vi "Forno USB.vi"() -> ()   [LabVIEW 2011]
panel:
  out "Manual OFF":bool
  out "Manual ON":bool
  out "Power":dbl(slide) scale=0.0..100.0
  out "Isteresi %":dbl(knob) scale=0.0..10.0
  out "Set Point":dbl(knob) scale=0.0..200.0
  out "Secondi":u8
  out "Minuti":u8
  out "Ora":u8
  in  "Timer ON-OFF":bool
  out "Tempo di funzionamento":cluster{dbl, dbl, dbl}(knob)={0.0, 1.0235355842339904, 13.033095966579117} scale=0.0..60.0
  in  "Secondi":u8(knob) scale=0.0..60.0
  in  "Minuti":u8(knob) scale=0.0..60.0
  in  "Ore":u8(knob) scale=0.0..24.0
  out "Orario":timestamp
  out "Temperatura Interna":dbl(slide) scale=0.0..300.0
  in  "On - Off":bool
  in  "Salvataggio Manuale":bool
  out "File salvato:":path
  in  "Nome File":string
  out "Grafico":cluster{dbl, dbl, dbl, dbl}(graph)
  out "Errore":bool
  out "Forno":bool
  # "DIG-0"
  # "DIG-1"
  # "Analog Channel 9"
  # "Analog Channel  8"
  # "Analog Channel 10"
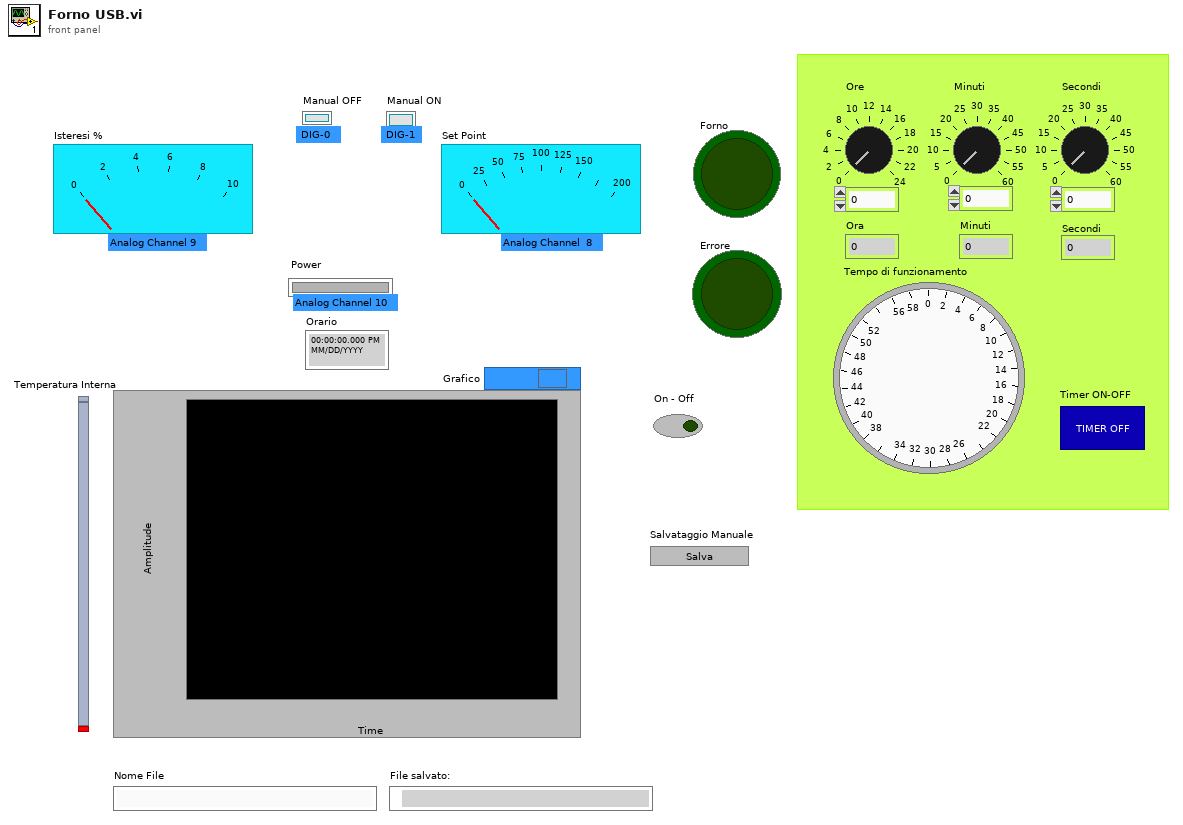
[diagram p1: front panel]
types:
  T1 = enum16{"open", "replace", "create", "open or create", "replace or create", "replace or create with confirmation"}
  T2 = typedef "LVDateTimeRec.ctl" = cluster{"fractional second":dbl, "second":i32, "minute":i32, "hour":i32, "day of month":i32, "month":i32, "year":i32, "day of week":i32, "day of year":i32, "DST":i32}
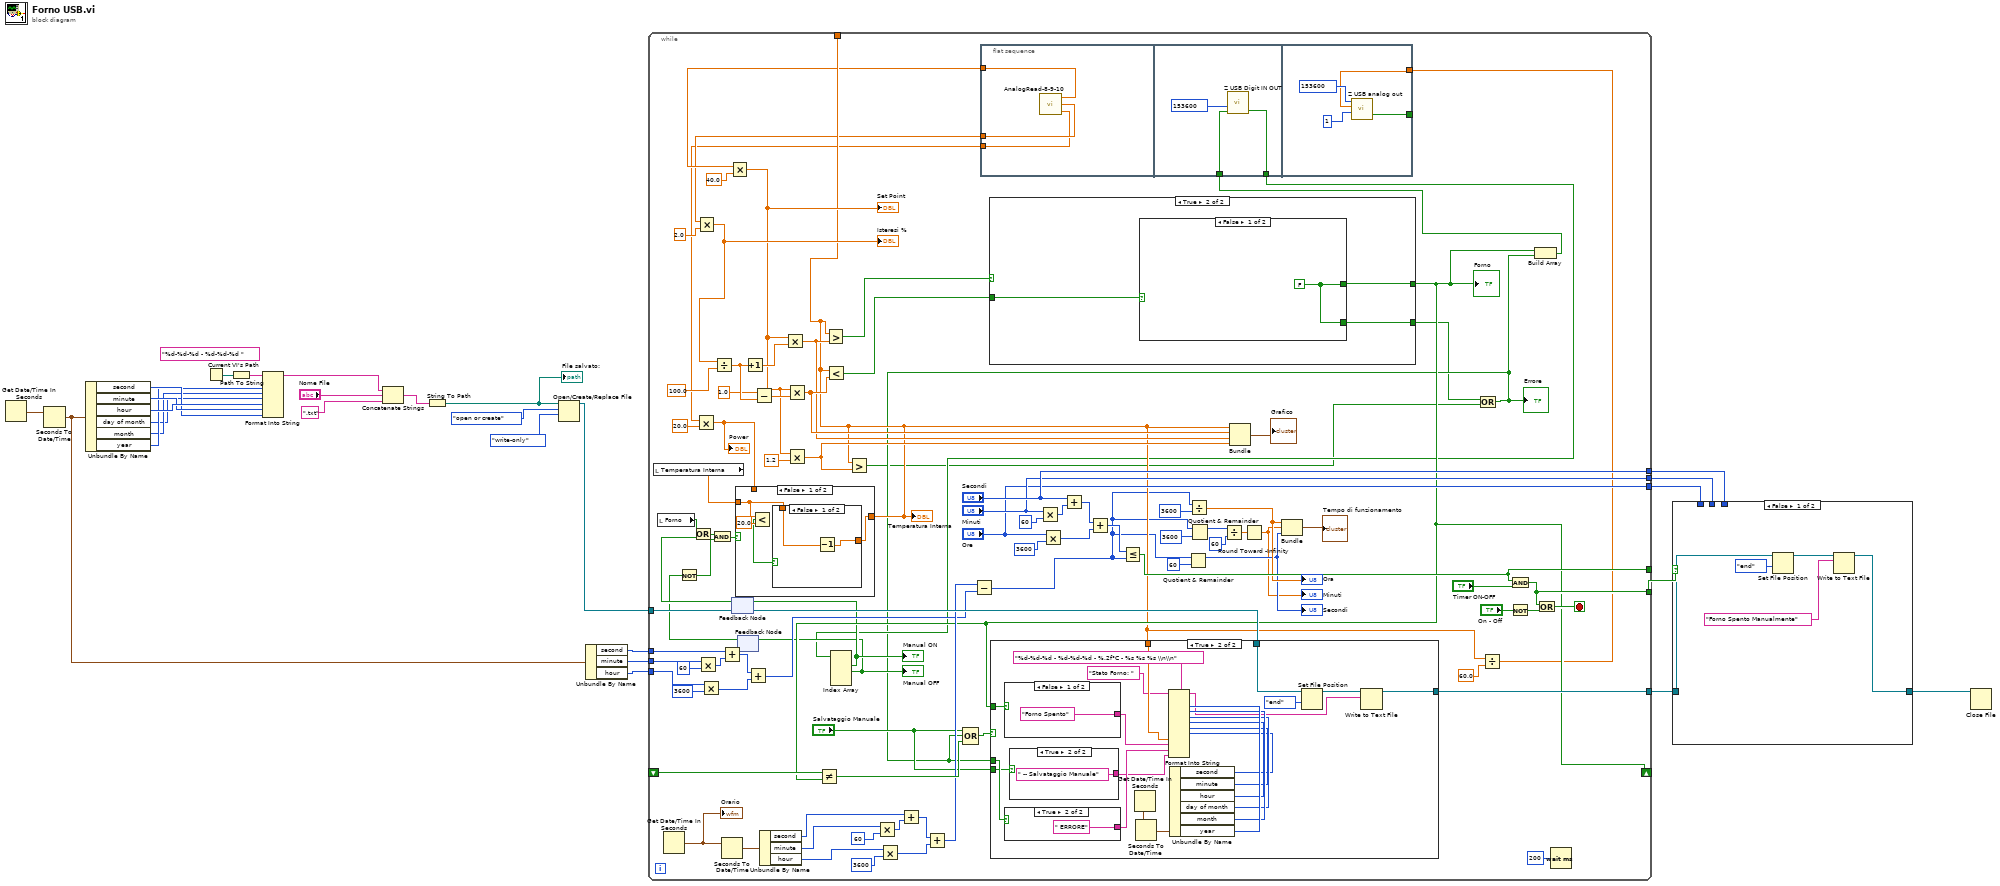
[diagram p0: block diagram]
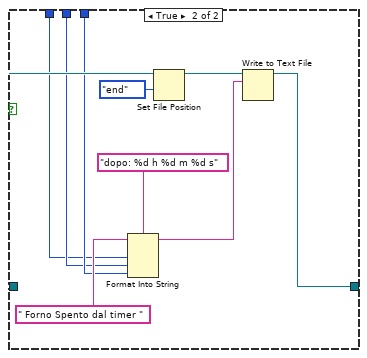
[diagram p2: hidden frame]
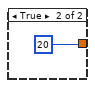
[diagram p3: hidden frame]
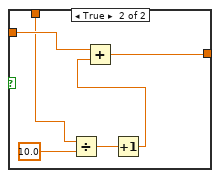
[diagram p4: hidden frame]
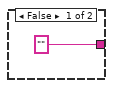
[diagram p6: hidden frame]
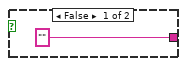
[diagram p7: hidden frame]
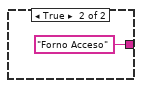
[diagram p8: hidden frame]
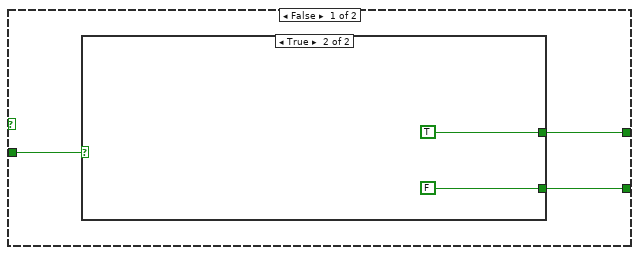
[diagram p9: hidden frame]
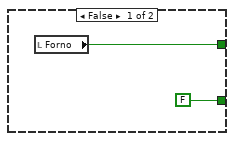
[diagram p10: hidden frame]
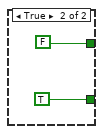
[diagram p11: hidden frame]
diagram:
  (unwired) "%d-%d-%d - %d-%d-%d " ("format string")
  n1 = Get Date/Time In Seconds() -> (seconds since 1Jan1904=w23:timestamp)
  n2 = Seconds To Date/Time(time stamp (now)=w23) -> (date time rec=w12:T2)  [unwired: 1 in]
  n3 = Unbundle By Name(w12) -> ("second"=w20:i32, "minute"=w21:i32, "hour"=w22:i32, "day of month"=w13:i32, "month"=w14:i32, "year"=w15:i32)
  n4 = Current VI's Path() -> (path=w2:path)
  n5 = Path To String(path=w2) -> (string=w1:string)
  n6 = Format Into String(initial string=w1, w15, w14, w13, w22, w21, w20) -> (resulting string=w19:string)  [unwired: 2 in, 1 out]
  n7 = Concatenate Strings(w19, "Nome File", ".txt" ("string")) -> (w25:string)
  n8 = String To Path(string=w25) -> (path=w24:path)
  "File salvato:" <- w24
  n9 = Open/Create/Replace File(file path (use dialog)=w24, operation (0:open)=T1."open or create", access (0:read/write)=enum16{"read/write", "read-only", "write-only"}."write-only") -> (refnum out=w16:refnum<file>)  [unwired: 3 in, 2 out]
  n10 = Unbundle By Name(w12) -> ("second"=w11:i32, "minute"=w10:i32, "hour"=w9:i32)
  n11 = while {
    tunnel: w16 -> [w105]
    tunnel: [w104] -> w8
    tunnel: [w49] -> _
    shift-right: [w55] -> _
    shift-left: _ -> [w100]
    tunnel: w11 -> [w97]
    tunnel: w10 -> [w96]
    tunnel: w9 -> [w93]
    tunnel: [w69] -> _
    tunnel: ["Secondi"] -> w6
    tunnel: ["Minuti"] -> w5
    tunnel: ["Ore"] -> w4
    tunnel: [w67] -> w3
    stop <- w74 stop-if-true
    n12 = local read "Temperatura Interna"() -> (w102:dbl)
    n13 = local read "Forno"() -> (w65:bool)
    n14 = Get Date/Time In Seconds() -> (seconds since 1Jan1904=w99:timestamp)
    "Orario" <- w99
    n15 = Multiply(x=w46, y=20.0) -> (x*y=w56:dbl)
    "Power" <- w56
    n16 = Multiply(x=w47, y=2.0) -> (x*y=w59:dbl)
    "Isteresi %" <- w59
    n17 = Multiply(x=w96, y=60) -> (x*y=w95:i32)
    n18 = Multiply(x=w93, y=3600) -> (x*y=w90:i32)
    n19 = Divide(x=w59, y=100.0) -> (x/y=w117:dbl)
    n20 = Add(x=w97, y=w95) -> (x+y=w91:i32)
    n21 = Seconds To Date/Time(time stamp (now)=w99) -> (date time rec=w98:T2)  [unwired: 1 in]
    n22 = Multiply(x=w48, y=40.0) -> (x*y=w58:dbl)
    "Set Point" <- w58
    n23 = feedback #1() -> (w54:bool)  [unwired: 1 in]
    n24 = Or(x=w65, y=w54) -> (x .or. y?=w64:bool)
    n25 = feedback #2() -> (w53:bool)  [unwired: 1 in]
    n26 = Not(x=w53) -> (.not. x?=w62:bool)
    n27 = And(x=w64, y=w62) -> (x .and. y?=w63:bool)
    n28 = case shown="False" w63 {
      tunnel: [w130 w142] -> w49
      tunnel: w102 -> [w131 w141]
      tunnel: w56 -> [_ w140]
      frame False {
        n29 = Less?(x=w131, y=20.0) -> (x < y?=w132:bool)
        n30 = case shown="False" w132 {
          tunnel: w131 -> [w135 _]
          tunnel: [w134 20] -> w130
          frame False {
            n31 = Decrement(x=w135) -> (x-1=w134:dbl)
          }
          frame True {
          }
        }
      }
      frame True {
        n32 = Divide(x=w140, y=10.0) -> (x/y=w138:dbl)
        n33 = Increment(x=w138) -> (x+1=w137:dbl)
        n34 = Add(x=w141, y=w137) -> (x+y=w142:dbl)
      }
    }
    "Temperatura Interna" <- w49
    n35 = Increment(x=w117) -> (x+1=w118:dbl)
    n36 = Add(x=w91, y=w90) -> (x+y=w80:i32)
    n37 = Subtract(x=1.0, y=w117) -> (x-y=w115:dbl)
    n38 = Unbundle By Name(w98) -> ("second"=w82:i32, "minute"=w83:i32, "hour"=w84:i32)
    n39 = Multiply(x=w58, y=w118) -> (x*y=w111:dbl)
    n40 = Multiply(x=w58, y=w115) -> (x*y=w112:dbl)
    n41 = Multiply(x=w58, y=1.2) -> (x*y=w107:dbl)
    n42 = Greater?(x=w49, y=w111) -> (0:w114:bool)
    n43 = Less?(x=w49, y=w112) -> (x < y?=w113:bool)
    n44 = Index Array(array=w44) -> (element #1=w52:bool, element #2=w51:bool)  [unwired: 4 in, 2 out]
    "Manual ON" <- w52
    "Manual OFF" <- w51
    n45 = feedback-in #1(w52) -> ()
    n46 = feedback-in #2(w51) -> ()
    n47 = Greater?(x=w49, y=w107) -> (0:w28:bool)
    n48 = Multiply(x=w83, y=60) -> (x*y=w89:i32)
    n49 = Multiply(x=w84, y=3600) -> (x*y=w85:i32)
    n50 = Add(x=w82, y=w89) -> (x+y=w86:i32)
    n51 = Add(x=w86, y=w85) -> (x+y=w81:i32)
    n52 = Subtract(x=w81, y=w80) -> (x-y=w36:i32)
    n53 = flat-sequence {
      tunnel: [w122] -> w48
      tunnel: [w121] -> w47
      tunnel: [w120] -> w46
      tunnel: w45 -> [w124]
      tunnel: [w123] -> w44
      tunnel: w43 -> [w127]
      tunnel: [w126] -> _
      frame #0 {
        n54 = call "AnalogRead-8-9-10.vi"() -> ("Ch 10"=w120:dbl, "Ch 9"=w121:dbl, "Ch 8"=w122:dbl)  [unwired: 3 out]
      }
      frame #1 {
        w125 = u32 153600 items=["9600"=9600, "19200"=19200, "38400"=38400, "76200"=76200, "153600"=153600, "307200"=307200, "614400"=614400, "1228800"=1228800] ("Baud Rate Asyn. Bit Bang")
        n55 = call "Z USB Digit IN OUT.vi"("Baud Rate Asyn. Bit Bang"=w125, "Uscite"=w124) -> ("Ingressi"=w123:bool[])  [unwired: 3 in, 2 out]
      }
      frame #2 {
        w128 = u32 153600 items=["9600"=9600, "19200"=19200, "38400"=38400, "76200"=76200, "153600"=153600, "307200"=307200, "614400"=614400, "1228800"=1228800] ("Baud Rate Asyn. Bit Bang")
        n56 = call "Z USB analog out.vi"("N° Channel"=i8 1, "V out"=w127, "Baud Rate Asyn. Bit Bang"=w128) -> ("USB error"=w126:bool)  [unwired: 1 in, 1 out]
      }
    }
    n57 = case shown="True" w114 {
      tunnel: w113 -> [w172 w181]
      tunnel: [w174 w179] -> w55
      tunnel: [w173 w180] -> w29
      frame False {
        n58 = case shown="True" w172 {
          tunnel: [w176 TRUE] -> w174
          tunnel: [FALSE FALSE] -> w173
          frame False {
            n59 = local read "Forno"() -> (w176:bool)
          }
          frame True {
          }
        }
      }
      frame True {
        n60 = case shown="False" w181 {
          tunnel: [w182 TRUE] -> w180
          tunnel: [w182 FALSE] -> w179
          frame False {
            w182 = FALSE
          }
          frame True {
          }
        }
      }
    }
    "Forno" <- w55
    n61 = Not Equal?(x=w100, y=w55) -> (x != y?=w101:bool)
    n62 = Multiply(x="Minuti", y=60) -> (x*y=w79:i32)
    n63 = Multiply(x="Ore", y=3600) -> (x*y=w75:i32)
    n64 = Add(x="Secondi", y=w79) -> (x+y=w76:i32)
    n65 = Add(x=w76, y=w75) -> (x+y=w40:i32)
    n66 = Less Or Equal?(x=w40, y=w36) -> (x <= y?=w69:bool)
    n67 = Quotient & Remainder(x=w36, y=60) -> (x-y*floor(x/y)=w38:i32)  [unwired: 1 out]
    "Secondi" <- w38
    n68 = Divide(x=w36, y=3600) -> (x/y=w39:dbl)
    "Ora" <- w39
    n69 = Quotient & Remainder(x=w36, y=3600) -> (x-y*floor(x/y)=w34:i32)  [unwired: 1 out]
    n70 = Divide(x=w34, y=60) -> (x/y=w32:dbl)
    n71 = Bundle(w49, w112, w111, w107) -> (→"Grafico":cluster{dbl, dbl, dbl, dbl})  [unwired: 1 in]
    n72 = Round Toward -Infinity(1:w32) -> (0:w31:dbl)
    "Minuti" <- w31
    n73 = Bundle(w39, w31, w38) -> (→"Tempo di funzionamento":cluster{dbl, dbl, i32})  [unwired: 1 in]
    n74 = Compound Arithmetic op=OR(w29, w28) -> (w30:bool)
    "Errore" <- w30
    n75 = Compound Arithmetic op=OR("Salvataggio Manuale", w30, w101) -> (w106:bool)
    n76 = case shown="True" w106 {
      tunnel: w30 -> [_ w147]
      tunnel: w55 -> [_ w151]
      tunnel: w105 -> [w143 w157]
      tunnel: [w143 w154] -> w104
      tunnel: w49 -> [_ w152]
      tunnel: "Salvataggio Manuale" -> [_ w145]
      frame False {
      }
      frame True {
        n77 = case shown="False" w151 {
          tunnel: ["Forno Spento" "Forno Acceso"] -> w149
          frame False {
          }
          frame True {
          }
        }
        n78 = case shown="True" w147 {
          tunnel: ["" " ERRORE"] -> w146
          frame False {
          }
          frame True {
          }
        }
        n79 = case shown="True" w145 {
          tunnel: ["" " -- Salvataggio Manuale"] -> w144
          frame False {
          }
          frame True {
          }
        }
        n80 = Get Date/Time In Seconds() -> (seconds since 1Jan1904=w150:timestamp)
        n81 = Seconds To Date/Time(time stamp (now)=w150) -> (date time rec=w159:T2)  [unwired: 1 in]
        n82 = Unbundle By Name(w159) -> ("second"=w160:i32, "minute"=w161:i32, "hour"=w162:i32, "day of month"=w163:i32, "month"=w164:i32, "year"=w165:i32)
        n83 = Format Into String "Format Into String"(format string="%d-%d-%d - %d-%d-%d - %.2f°C - %s %s %s \\n\\n", initial string="Stato Forno: ", w165, w164, w163, w162, w161, w160, w152, w149, w146, w144) -> (resulting string=w153:string)  [unwired: 1 in, 1 out]
        n84 = Set File Position(refnum=w157, from (0:start)=enum16{"start", "end", "current"}."end") -> (refnum out=w155:refnum<file>)  [unwired: 2 in, 1 out]
        n85 = Write to Text File(file (use dialog)=w155, text=w153) -> (refnum out=w154:refnum<file>)  [unwired: 2 in, 2 out]
      }
    }
    n86 = Divide(x=w49, y=60.0) -> (x/y=w43:dbl)
    n87 = And(x=w69, y="Timer ON-OFF") -> (x .and. y?=w67:bool)
    n88 = Not(x="On - Off") -> (.not. x?=w70:bool)
    n89 = Build Array(w55, w30) -> (w45:bool[])
    n90 = Or(x=w67, y=w70) -> (x .or. y?=w74:bool)
    n91 = Wait (ms)(milliseconds to wait=u32 200) -> ()  [unwired: 1 out]
  }
  n92 = case shown="False" w3 {
    tunnel: w8 -> [w185 w196]
    tunnel: [w186 w197] -> w7
    tunnel: w6 -> [_ w192]
    tunnel: w5 -> [_ w191]
    tunnel: w4 -> [_ w190]
    frame False {
      n93 = Set File Position(refnum=w185, from (0:start)=enum16{"start", "end", "current"}."end") -> (refnum out=w188:refnum<file>)  [unwired: 2 in, 1 out]
      n94 = Write to Text File(file (use dialog)=w188, text="Forno Spento Manualmente") -> (refnum out=w186:refnum<file>)  [unwired: 2 in, 2 out]
    }
    frame True {
      n95 = Format Into String "Format Into String"(format string="dopo: %d h %d m %d s", initial string=" Forno Spento dal timer ", w190, w191, w192) -> (resulting string=w195:string)  [unwired: 1 in, 1 out]
      n96 = Set File Position(refnum=w196, from (0:start)=enum16{"start", "end", "current"}."end") -> (refnum out=w198:refnum<file>)  [unwired: 2 in, 1 out]
      n97 = Write to Text File(file (use dialog)=w198, text=w195) -> (refnum out=w197:refnum<file>)  [unwired: 2 in, 2 out]
    }
  }
  n98 = Close File(refnum=w7) -> ()  [unwired: 1 in, 2 out]
